vi "LUCS001RT_GPS_UBX_ReceiverRev5.vi"(8 "error in":errorcluster, 10 "FPGA VI Reference":refnum<k20>, 11 "GPS DataIn":T1 {"UTC Valid" items=["UTC not valid", "Valid Time of Week", "Valid Week Number", "NA", "Valid UTC"]; "CAcc" format="%.0f°"; "Heading(2-D)" format="%0.6f°"; "GSpeed(2-D)" format="%.0f cm/s"; "Speed(3-D)" format="%.0f cm/s"; "NED_DNvsty" format="%.0f cm/s"; "NED_Evsty" format="%.0f cm/s"; "NED_NVsty" format="%.0f cm/s"; "Sacc" format="%.0f cm/s"; "ECEF_Z_Vlsty" format="%.0f cm/s"; "ECEF_Y_Vlsty" format="%.0f cm/s"; "ECEF_X_Vlsty" format="%.0f cm/s"; "FixType" items=["No Fix", "Dead Reckoning Only", "2D-Fix", "3D-Fix", "GPS + Dead Reckoning", "Time Only Fix", "RESERVED"]; "Vacc" format="%.0f mm"; "Hacc" format="%.0f mm"; "HMSL" format="%d mm"; "HEIGHT" format="%.0f mm"; "LAT" format="%#.6f"; "LON" format="%#.6f"; "Waypoint:XTE" format="%#.2f"}) -> (0 "error out":errorcluster, 3 "GPS Data Out":T1 {"UTC Valid" items=["UTC not valid", "Valid Time of Week", "Valid Week Number", "NA", "Valid UTC"]; "CAcc" format="%.0f°"; "Heading(2-D)" format="%0.6f°"; "GSpeed(2-D)" format="%.0f cm/s"; "Speed(3-D)" format="%.0f cm/s"; "NED_DNvsty" format="%.0f cm/s"; "NED_Evsty" format="%.0f cm/s"; "NED_NVsty" format="%.0f cm/s"; "Sacc" format="%.0f cm/s"; "ECEF_Z_Vlsty" format="%.0f cm/s"; "ECEF_Y_Vlsty" format="%.0f cm/s"; "ECEF_X_Vlsty" format="%.0f cm/s"; "FixType" items=["No Fix", "Dead Reckoning Only", "2D-Fix", "3D-Fix", "GPS + Dead Reckoning", "Time Only Fix", "RESERVED"]; "Vacc" format="%.0f mm"; "Hacc" format="%.0f mm"; "HMSL" format="%d mm"; "HEIGHT" format="%.0f mm"; "LAT" format="%#.6f"; "LON" format="%#.6f"; "Waypoint:XTE" format="%#.2f"}, 4 "FullGPS Message":u8[](array[numeric]) format="%02x", 6 "GPS.DataReceived":bool)   [LabVIEW 2020]
uses:
  LUCS001RT_GPS_Data.ctl
panel:
  # "WAYPOINT"
  # "CURRENT POSITION"
  # "WAYPOINT"
  # "CURRENT POSITION"
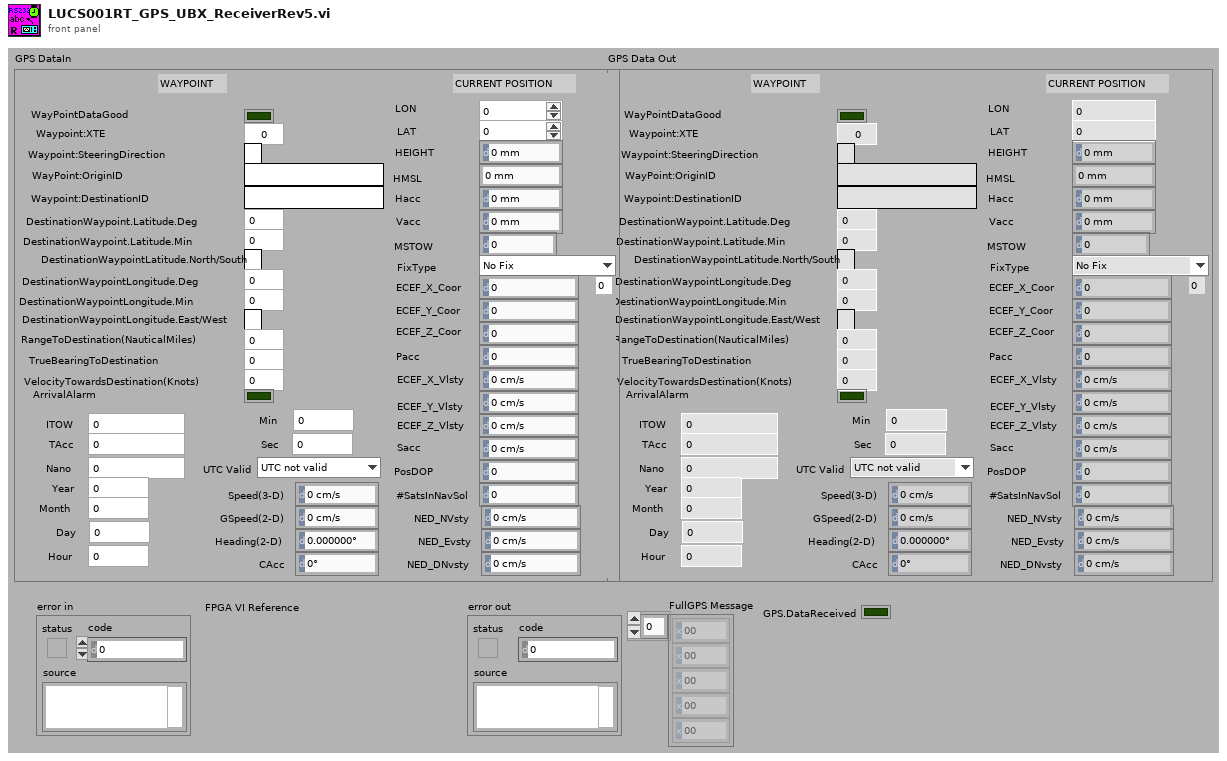
[diagram p1: front panel]
types:
  T1 = typedef "LUCS001RT_GPS_Data.ctl" = cluster{"WayPointDataGood":bool, "Waypoint:XTE":dbl, "Waypoint:SteeringDirection":string, "WayPoint:OriginID":string, "Waypoint:DestinationID":string, "DestinationWaypoint.Latitude.Deg":i32, "DestinationWaypoint.Latitude.Min":dbl, "DestinationWaypointLatitude.North/South":string, "DestinationWaypointLongitude.Deg":i32, "DestinationWaypointLongitude.Min":dbl, "DestinationWaypointLongitude.East/West":string, "RangeToDestination(NauticalMiles)":dbl, "TrueBearingToDestination":dbl, "VelocityTowardsDestination(Knots)":dbl, "ArrivalAlarm":bool, "ITOW":u32, "TAcc":u32, "LON":dbl, "LAT":dbl, "HEIGHT":i32, "HMSL":i32, "Hacc":u32, "Vacc":u32, "MSTOW":u32, "FixType":u8, "ECEF_X_Coor":i32, "ECEF_Y_Coor":i32, "ECEF_Z_Coor":i32, "Pacc":u32, "ECEF_X_Vlsty":i32, "ECEF_Y_Vlsty":i32, "ECEF_Z_Vlsty":i32, "Sacc":u32, "PosDOP":u16, "#SatsInNavSol":u8, "NED_NVsty":i32, "NED_Evsty":i32, "NED_DNvsty":i32, "Speed(3-D)":u32, "GSpeed(2-D)":u32, "Heading(2-D)":dbl, "CAcc":u32, "Nano":i32, "Year":u16, "Month":u8, "Day":u8, "Hour":u8, "Min":u8, "Sec":u8, "UTC Valid":u8}
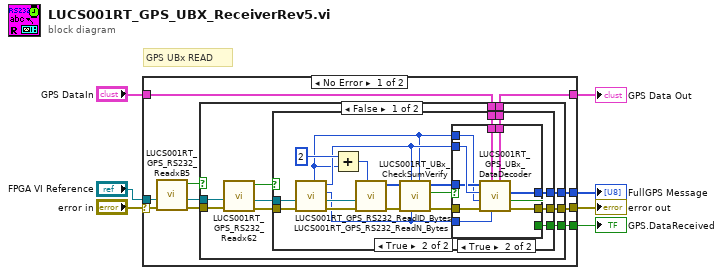
[diagram p0: block diagram]
diagram:
  # "GPS UBx READ"
  n1 = case shown="No Error" "error in" {
    selector: "error in" -> [w17 w63]
    tunnel: [w10 w63] -> w6
    tunnel: "FPGA VI Reference" -> [w16 _]
    tunnel: "GPS DataIn" -> [w15 _]
    tunnel: [w14 _] -> w4
    tunnel: [w9 _] -> w3
    tunnel: [w8 _] -> w2
    frame No Error {
      n2 = call "LUCS001RT_GPS_RS232_ReadxB5.vi"("error in"=w17, "FPGA VI Reference"=w16) -> ("error out"=w13:errorcluster, "FPGA VI Reference Out"=w11:refnum<k20>, "TimedOut?"=w12:bool)  [unwired: 7 out]
      n3 = case shown="False" w12 {
        tunnel: w13 -> [w27 w62]
        tunnel: w11 -> [w22 _]
        tunnel: [w23 w62] -> w10
        tunnel: w15 -> [w21 w61]
        tunnel: [w20 w61] -> w14
        tunnel: [w19 _] -> w9
        tunnel: [w18 _] -> w8
        frame False {
          n4 = call "LUCS001RT_GPS_RS232_Readx62.vi"("error in"=w27, "FPGA VI Reference In"=w22) -> ("error out"=w26:errorcluster, "FPGA VI Reference Out"=w25:refnum<k20>, "x62?"=w24:bool)  [unwired: 7 out]
          n5 = case shown="True" w24 {
            tunnel: w26 -> [w29 w48]
            tunnel: w25 -> [_ w47]
            tunnel: [w29 w39] -> w23
            tunnel: w21 -> [w28 w36]
            tunnel: [w28 w35] -> w20
            tunnel: [_ w32] -> w19
            tunnel: [_ w31] -> w18
            frame False {
            }
            frame True {
              n6 = call "LUCS001RT_GPS_RS232_ReadID_Bytes.vi"("error in"=w48, "FPGA VI Reference"=w47) -> ("error out"=w46:errorcluster, "FPGA VI Reference Out"=w45:refnum<k20>, "ID"=w34:u8, "Class"=w38:u8, "Length"=w30:u16)  [unwired: 5 out]
              n7 = Add(x=u16 2, y=w30) -> (x+y=w44:u16)
              n8 = call "LUCS001RT_GPS_RS232_ReadN_Bytes.vi"("NumberOfBytesToRead"=w44, "error in"=w46, "FPGA VI Reference"=w45) -> ("error out"=w42:errorcluster, "N-BytesOut"=w33:u8[])  [unwired: 7 out]
              n9 = call "LUCS001RT_UBx_CheckSumVerify.vi"("Length"=w30, "ID"=w34, "Class"=w38, "error in (no error)"=w42, "N-Bytes"=w33) -> ("error out"=w41:errorcluster, "CheckSumOK?"=w40:bool, "N-BytesDUP"=w37:u8[])  [unwired: 1 in, 3 out]
              n10 = case shown="True" w40 {
                tunnel: w41 -> [w50 w59]
                tunnel: [w50 w57] -> w39
                tunnel: w38 -> [_ w60]
                tunnel: w34 -> [_ w58]
                tunnel: w37 -> [_ w52]
                tunnel: w36 -> [w49 w54]
                tunnel: [w49 w53] -> w35
                tunnel: [_ w56] -> w32
                tunnel: [_ w55] -> w31
                tunnel: w30 -> [_ w51]
                frame False {
                }
                frame True {
                  n11 = call "LUCS001RT_GPS_UBx_DataDecoder.vi"("ID"=w58, "GPS DataIn"=w54, "error in"=w59, "Length"=w51, "Class"=w60, "N-BytesIn"=w52) -> ("error out"=w57:errorcluster, "GPS.DataReceived"=w55:bool, "CompleteGPS_UBxMessageOut"=w56:u8[], "GPS DataOut"=w53:T1)  [unwired: 2 out]
                }
              }
            }
          }
        }
        frame True {
        }
      }
    }
    frame Error {
    }
  }
  "error out" <- w6
  "GPS Data Out" <- w4
  "FullGPS Message" <- w3
  "GPS.DataReceived" <- w2
